vi "PathDrawerMain.vi"() -> ()   [LabVIEW 2017]
uses:
  Shared/PathFileData.ctl
  Shared/RobotNeededPathData.ctl
panel:
  in  "Tab Control":enum32{"Path", "Load/Save"}(tab)
  in  "SlowSpeed":dbl=15.0 format="%#_13g"
  in  "SlowDistanceAtEnd":dbl=12.0 format="%#_13g"
  in  "Speed/Curve":dbl=2.0 format="%#_13g"
  in  "DriveBackwards?":bool
  in  "Lookahead":dbl=13.0
  out "Points (in)":cluster{dbl, dbl}[](array[cluster])=[{14.875179340028694, 248.22955523672883}, {20.874656142200276, 248.30358846723587}, {26.874111844136586, 248.37762105138137}, {32.87350807743945, 248.45164576572313}, {38.87285031681461, 248.52564930010115}, {44.8721376174185, 248.59961966708173}, {50.87132679490307, 248.67354461649725}, {56.87033754344792, 248.74740402354425}, {62.86906734714655, 248.82116341910367}, {68.86738582507886, 248.8947700228471}, {74.8651048928512, 248.9681473786283}, {80.86193607975939, 249.04118420575625}, {86.85743425686633, 249.11371611190245}, {92.85096070503305, 249.18549244057994}, {98.84145913304778, 249.25615421906943}, {104.8276556156584, 249.32512066220386}, {110.80708687815371, 249.39160976611277}, {116.77680979233328, 249.4543515328238}, {122.73186791730424, 249.5115256430506}, {128.6649834222615, 249.56041338385793}, {134.56548779738634, 249.5969246365727}, {140.417375186257, 249.6149706245841}, {146.1966910294908, 249.60548863042237}, {151.86775390690585, 249.55495714900198}, {157.37740484291632, 249.4431992192172}, {162.64635606562646, 249.2401236836006}, {167.55632241578652, 248.9008602167623}, {172.80142342709613, 248.36924030479463}, {178.27099698643164, 247.70868036210402}, {183.89073844553332, 246.9617176111296}, {189.61066276690974, 246.15689887726526}, {195.3970009046773, 245.3134049055755}, {201.22672879119182, 244.44415649854506}, {207.08384341112958, 243.55790546653972}, {212.9567773862825, 242.6606503511154}, {218.83652869344567, 241.75660718632653}, {224.71520193237015, 240.84889249476205}, {230.58472714757215, 239.94002850052652}, {236.43555125878544, 239.03235181687802}, {242.25509137335504, 238.1283916506969}, {248.0256984324822, 237.231278977795}, {253.72180303927817, 236.34525315742894}, {259.30577066584806, 235.47634844945551}, {264.7218219756948, 234.63337048251796}, {269.8869762914892, 233.8293235417345}, {274.67764890352106, 233.08351364924852}, {278.909612625538, 232.42467718794836}]
  in  "Points":cluster{dbl, dbl}[](array[cluster])=[{40.0, 78.0}, {202.0, 76.0}, {324.0, 95.0}]
  in  "Roundedness":dbl(slide)=0.8606565656565657 scale=0.6..0.997
  in  "Length":dbl=38.5
  in  "Width":dbl=33.0
  in  "CenterRotOffset":dbl=15.5
  in  "PointSpacing":dbl=6.0 min=1.0 format="%#_13g"
  in  "Flip Path":bool
  in  "MaxVel":dbl=110.0 format="%#_13g"
  in  "MaxAccel":dbl=50.0 format="%#_13g"
  in  "StartingPosition":enum16{"1", "2", "3", "4", "No Preset"}(ring)
  in  "ExportAllToRobot":bool
  in  "LocalTempPaths":i32(listbox)
  out "standard output":string
  in  "SaveToLocal":bool
  in  "LoadFromLocal":bool
  in  "ExportToRobot":bool
  in  "LoadAllFromRobot":bool
  in  "LocalPaths":i32(listbox)=2
  out "standard error":string="NI Linux Real-Time (run mode)\n\nLog in with your NI-Auth credentials.\n\n"
  in  "LocalFileNames":string[](array[string])=["1A.txt", "1B.txt", "1C.txt", "1D.txt", "2A.txt", "2B.txt", "2C.txt", "2D.txt", "3A.txt", "3B.txt", "3C.txt", "3D.txt", "4A.txt", "4B.txt", "4C.txt", "4D.txt"]
  in  "Stop":bool
  out "Path Drawer":T1(plugin-control)
  # "Includes bumpers"
  # "INSTRUCTIONS"
  # "The red line is the path that the robot recieves. Everything else is to help create that path\n\nUse the multi-line tool to draw a path. Double click to stop drawing.\nHover over a node and press backspace to remove it.\nPress I to insert a new node (at the end of the path only, for now)\n\nUse the contols to input robot width, height, and center of rotation offset,\nHow far apart the points in the \"real world units\" path are,\nWhether the robot travels on the left or right of your green lines, and\nthe roundedness of the path. (Note: point spacing affects roundedness)\n\nYou can manually edit the green node's location in the path with the Points array,\nor drag the nodes on the image\n\nPress Export To File and enter the file name (no extension) to save the path to a file in the\nThisVIsDirectory\\Paths\\ folder\n\nIf you acidentally clear your path press Z quickly to get it back"
  # "Responses of CMDs run"
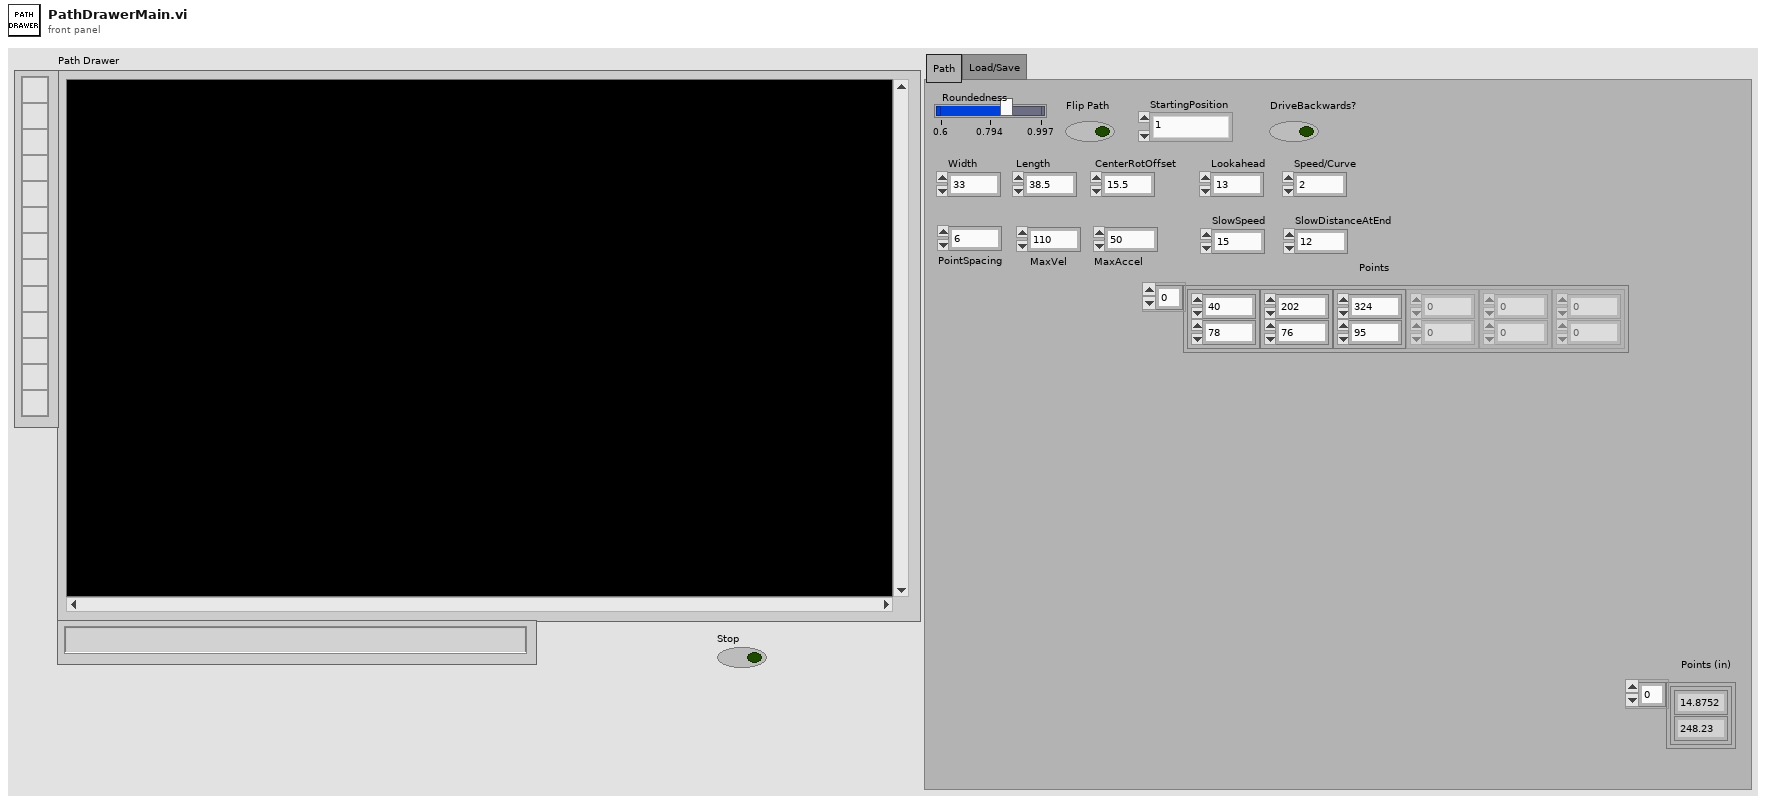
[diagram p1: front panel]
types:
  T1 = typedef "IMAQ Image.ctl" = refnum<image>
  T2 = typedef "Image Type" = u32
  T3 = enum16{"open", "replace", "create", "open or create", "replace or create", "replace or create with confirmation"}
  T4 = cluster{"Global Rectangle":i32[], "Contours":cluster{"Contour Type":u32, "ROI Type":u32, "Points":i32[]}[]}
  T5 = cluster{"Contour Type":u32, "ROI Type":u32, "Points":i32[]}[]
  T6 = cluster{"Contour Type":u32, "ROI Type":u32, "Points":i32[]}
  T7 = typedef "PathFileData.ctl" = cluster{"RobotNeeded":T8, "Meta":cluster{"Path (px)":cluster{i32, i32}[], "RobotWidth":dbl, "RobotLength":dbl, "CenterOfRotYOffset":dbl, "Roundedness":dbl, "StartingPositionPreset":u32, "PathName":string}}
  T8 = typedef "RobotNeededPathData.ctl" = cluster{"Path":cluster{dbl, dbl}[], "MaxVel":dbl, "MaxAccel":dbl, "Backwards?":bool, "PointSpacing":dbl, "LookaheadDist":dbl, "Speed/Curve":dbl, "SlowDistanceAtEnd":dbl, "SlowSpeed":dbl}
  T9 = cluster{"Path (px)":cluster{i32, i32}[], "RobotWidth":dbl, "RobotLength":dbl, "CenterOfRotYOffset":dbl, "Roundedness":dbl, "StartingPositionPreset":u32, "PathName":string}
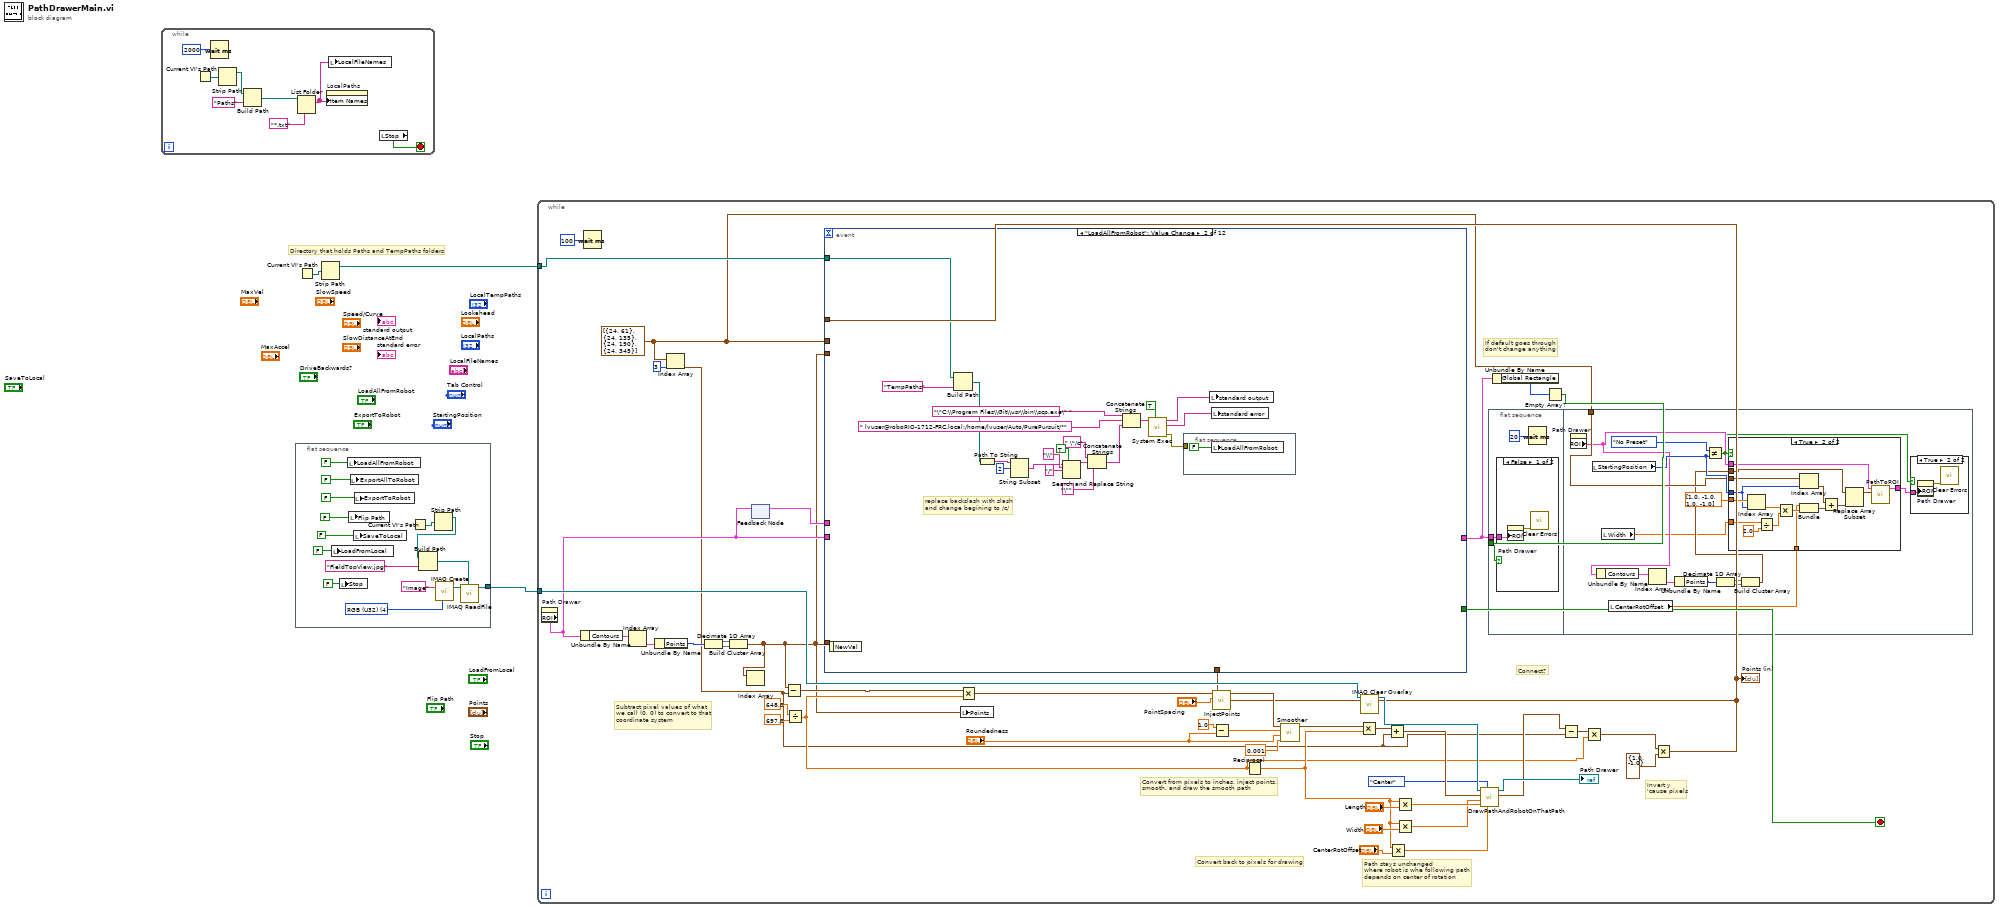
[diagram p0: block diagram]
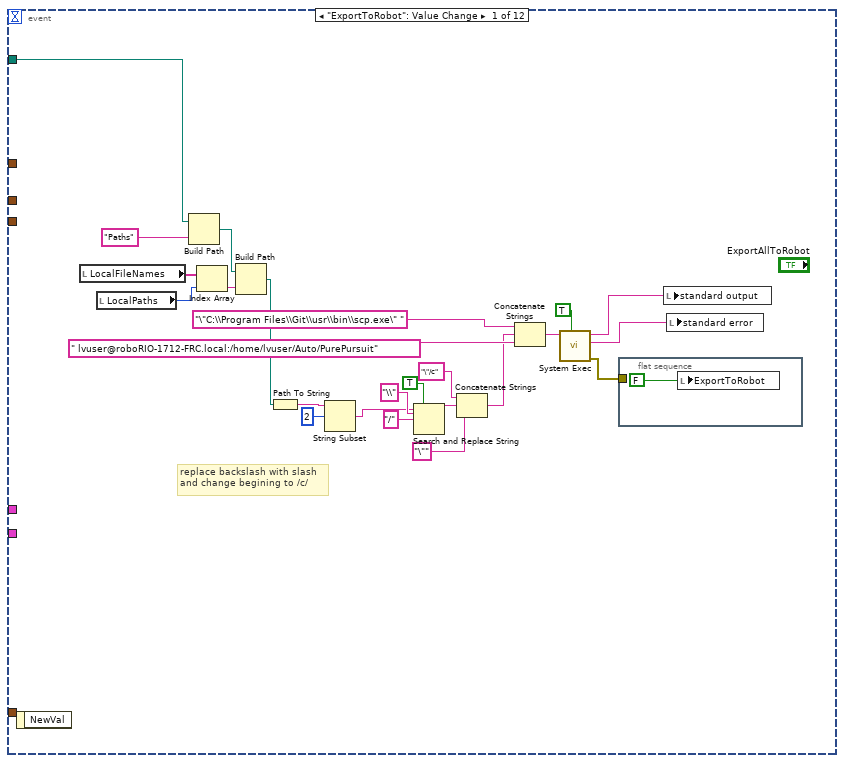
[diagram p5: hidden frame]
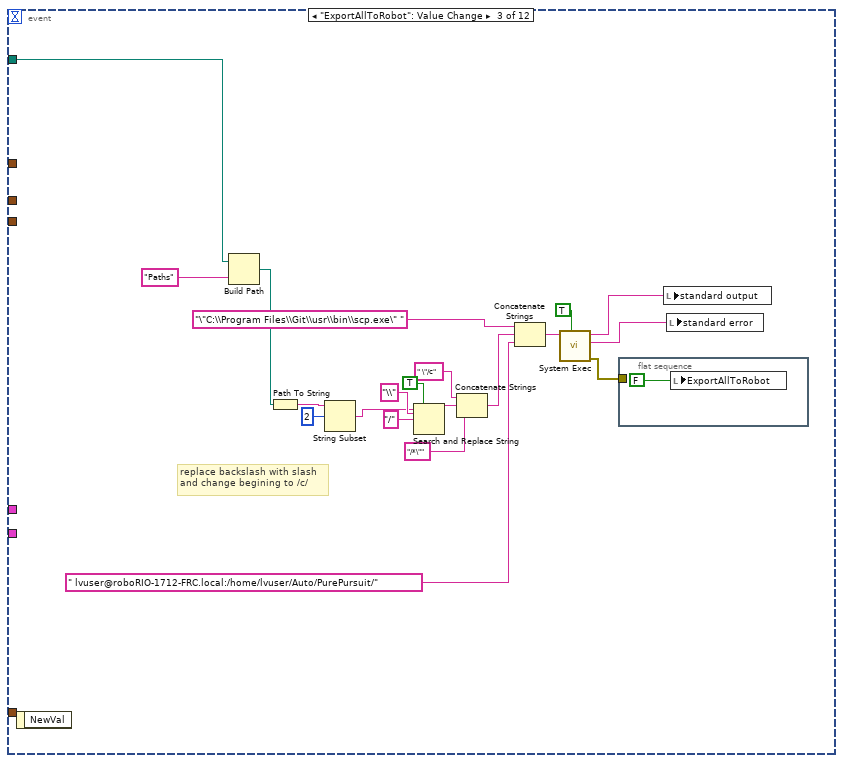
[diagram p6: hidden frame]
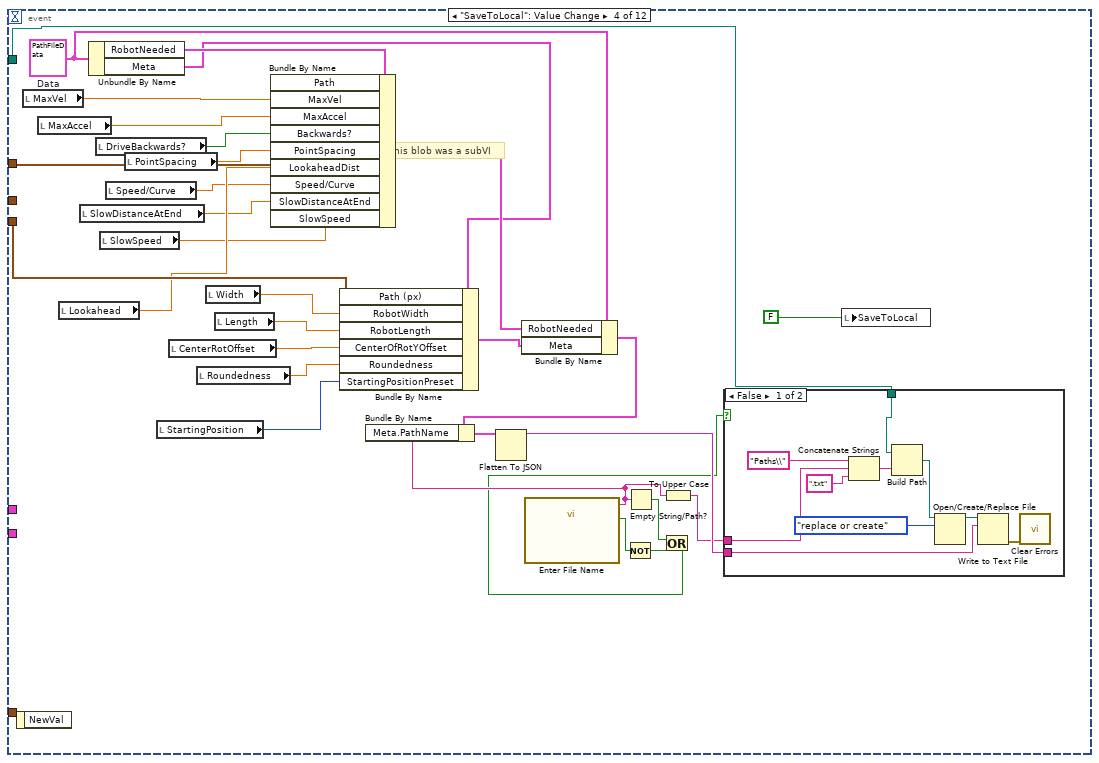
[diagram p7: hidden frame]
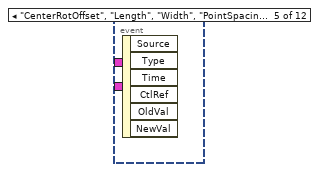
[diagram p9: hidden frame]
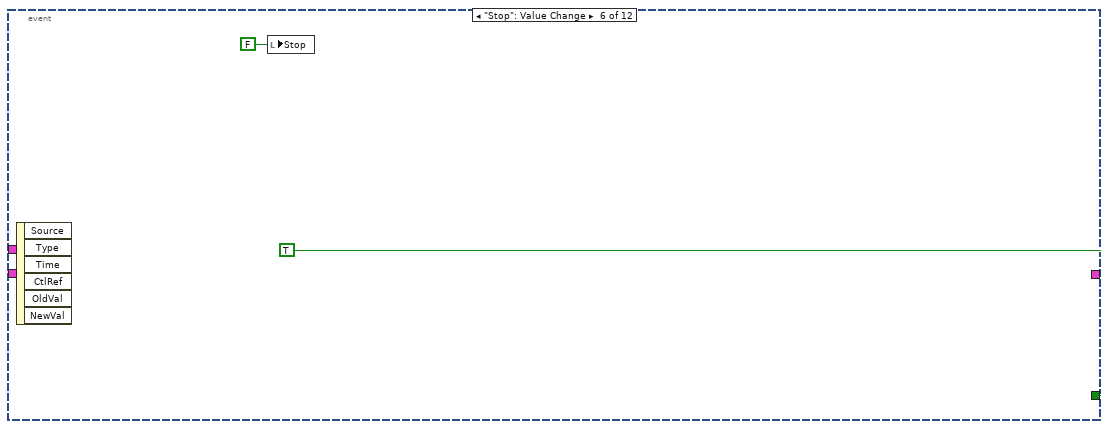
[diagram p10: hidden frame]
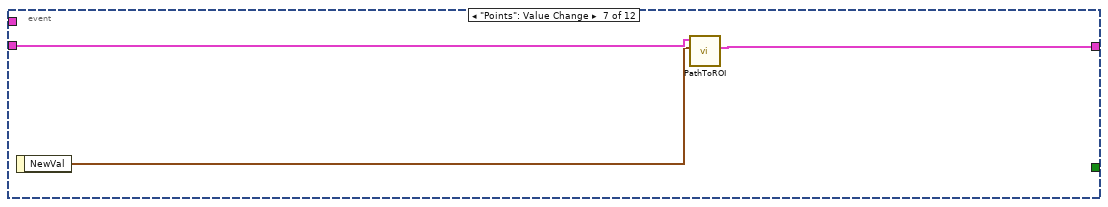
[diagram p11: hidden frame]
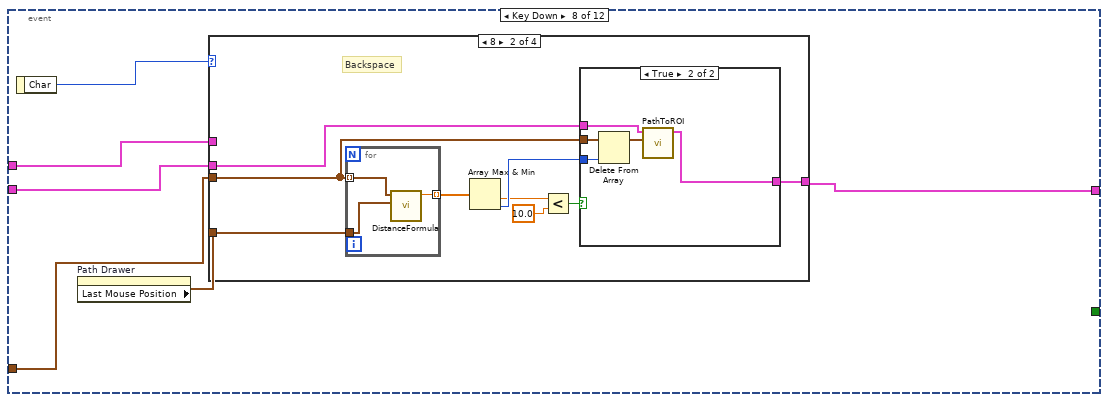
[diagram p12: hidden frame]
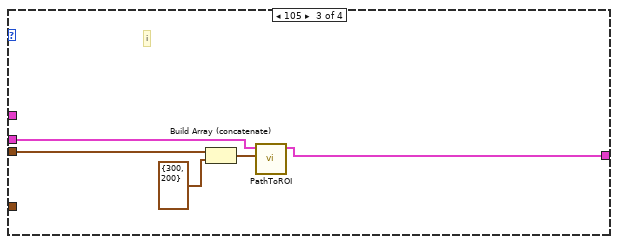
[diagram p15: hidden frame]
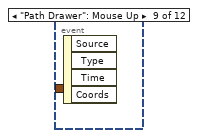
[diagram p17: hidden frame]
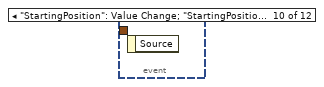
[diagram p18: hidden frame]
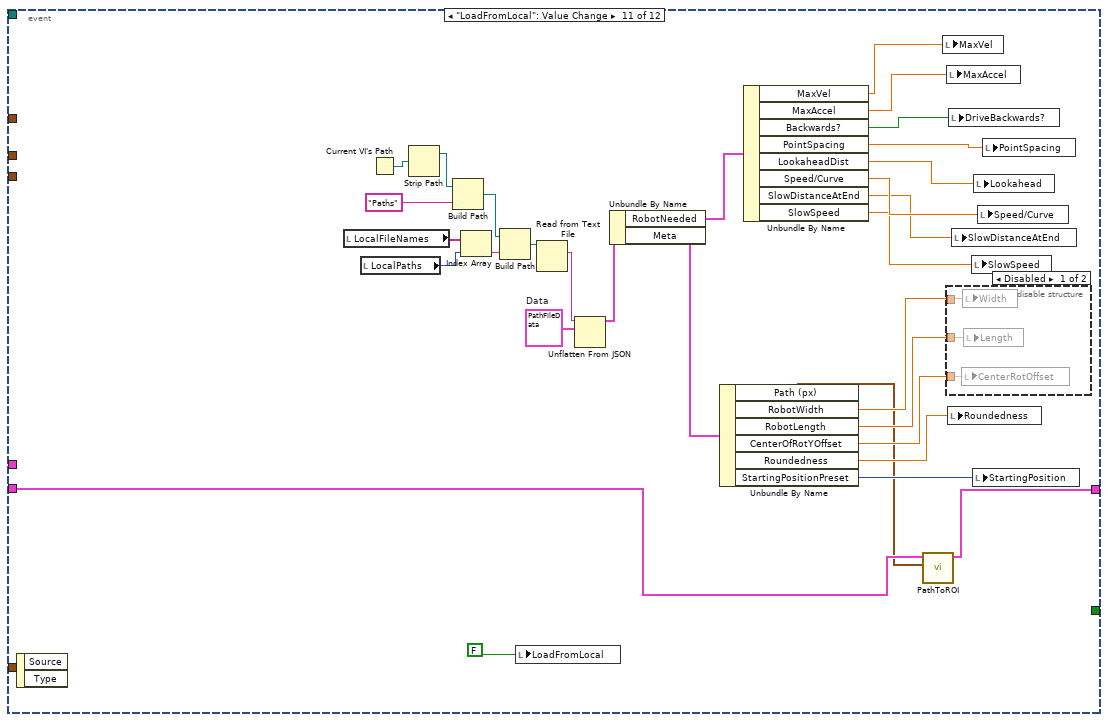
[diagram p19: hidden frame]
diagram:
  # "Directory that holds Paths and TempPaths folders"
  n1 = while {
    stop <- w10 stop-if-true
    n2 = Current VI's Path() -> (path=w5:path)
    n3 = Wait (ms)(milliseconds to wait=u32 2000) -> ()  [unwired: 1 out]
    n4 = Strip Path(path=w5) -> (stripped path=w4:path)  [unwired: 1 out]
    n5 = Build Path(base path=w4, name or relative path="Paths") -> (appended path=w7:path)
    n6 = List Folder(path=w7, pattern="*.txt") -> (filenames=w9:string[])  [unwired: 2 in, 3 out]
    n7 = property on="LocalPaths" class="LstBox (strict)"("Item Names"=w9) -> ()  [unwired: 2 in, 2 out]
    n8 = local write "LocalFileNames"(w9) -> ()
    n9 = local read "Stop"() -> (w10:bool)
  }
  n10 = flat-sequence {
    tunnel: [w21] -> w3
    frame #0 {
      w23 = T2 4 items=["Grayscale (U8)", "Grayscale (I16)", "Grayscale (SGL)", "Complex (CSG)", "RGB (U32)", "HSL (U32)", "RGB (U64)", "Grayscale (U16)"] ("Image Type")
      n11 = local write "LoadFromLocal"(FALSE ("Export To File")) -> ()
      n12 = local write "Stop"(FALSE ("Stop")) -> ()
      n13 = local write "LoadAllFromRobot"(FALSE ("Export To File")) -> ()
      n14 = local write "Flip Path"(FALSE ("Export To File")) -> ()
      n15 = local write "ExportAllToRobot"(FALSE ("Export To File")) -> ()
      n16 = local write "SaveToLocal"(FALSE ("Export To File")) -> ()
      n17 = local write "ExportToRobot"(FALSE ("Export To File")) -> ()
      n18 = Current VI's Path() -> (path=w15:path)
      n19 = Strip Path(path=w15) -> (stripped path=w14:path)  [unwired: 1 out]
      n20 = Build Path(base path=w14, name or relative path="FieldTopView.jpg") -> (appended path=w25:path)
      n21 = call "IMAQ Create"("Image Name"="Image", "Image Type"=w23) -> ("New Image"=w22:T1)  [unwired: 3 in, 1 out]
      n22 = call "IMAQ ReadFile"("File Path"=w25, "Image"=w22) -> ("Image Out"=w21:T1)  [unwired: 5 in, 4 out]
    }
  }
  n23 = Current VI's Path() -> (path=w2:path)
  n24 = Strip Path(path=w2) -> (stripped path=w1:path)  [unwired: 1 out]
  n25 = while {
    tunnel: w3 -> [w67]
    tunnel: w1 -> [w33]
    stop <- w41 stop-if-true
    w27 = cluster{i32, i32}[] [{24, 61}, {24, 135}, {24, 190}, {24, 345}]
    # "Connect?"
    # "Invert y\n'cause pixels"
    # "Path stays unchanged\nwhere robot is whe following path\ndepends on center of rotation"
    # "Convert back to pixels for drawing"
    # "If default goes through\ndon't change anything"
    # "Convert from pixels to inches, inject points,\nsmooth, and draw the smooth path"
    # "Subtract pixel values of what\nwe call (0, 0) to convert to that\ncoordinate system"
    n26 = property on="Path Drawer" class="ImageControl"() -> ("ROI"=w37:T4)  [unwired: 2 in, 2 out]
    n27 = Unbundle By Name(w37) -> ("Contours"=w73:T5)
    n28 = Wait (ms)(milliseconds to wait=u32 100) -> ()  [unwired: 1 out]
    n29 = Index Array(array=w73) -> (element=w68:T6)  [unwired: 1 in]
    n30 = Unbundle By Name(w68) -> ("Points"=w62:i32[])
    n31 = Index Array(array=w27, index=3) -> (element=w31:cluster{i32, i32})
    n32 = Decimate 1D Array(w62) -> (w72:i32[], w71:i32[])
    n33 = Build Cluster Array(w72, w71) -> (w35:cluster{i32, i32}[])
    n34 = Index Array(array=w35) -> ()  [unwired: 1 in, 1 out]
    n35 = feedback-in #1(w37) -> ()
    n36 = feedback #1() -> (w50:T4)  [unwired: 1 in]
    n37 = Subtract(x=w35, y=w31) -> (x-y=w63:cluster{i32, i32}[])
    n38 = Divide(x=648.0, y=697.0) -> (x/y=w38:dbl)
    n39 = Multiply(x=w63, y=w38) -> (x*y=w51:cluster{dbl, dbl}[])
    n40 = local write "Points"(w35) -> ()
    n41 = call "InjectPoints.vi"("Distance"="PointSpacing", "Path"=w51) -> ("Path out"=w65:cluster{dbl, dbl}[])  [unwired: 9 in]
    n42 = Subtract(x=1.0, y="Roundedness") -> (x-y=w60:dbl)
    n43 = Reciprocal(x=w38) -> (1/x=w48:dbl)
    n44 = call "Smoother.vi"("tolerance"=0.001, "B"="Roundedness", "A"=w60, "Path"=w65) -> ("SmoothPath"=w56:cluster{dbl, dbl}[])  [unwired: 7 in]
    n45 = Multiply(x=w56, y=w48) -> (x*y=w64:cluster{dbl, dbl}[])
    n46 = call "IMAQ Clear Overlay"("Image"=w67) -> ("Image Out"=w45:T1)  [unwired: 9 in, 1 out]
    n47 = Add(x=w64, y=w31) -> (x+y=w44:cluster{dbl, dbl}[])
    n48 = Multiply(x=w48, y="CenterRotOffset") -> (x*y=w28:dbl)
    n49 = Multiply(x=w48, y="Length") -> (x*y=w43:dbl)
    n50 = Multiply(x=w48, y="Width") -> (x*y=w29:dbl)
    n51 = call "DrawPathAndRobotOnThatPath.vi"("CenterOfRotYOffset (px)"=w28, "PathMode"=enum16{"Left", "Right", "Center"}."Center", "RobotLength (px)"=w43, "RobotWidth (px)"=w29, "Path (px)"=w44, "Image In"=w45) -> ("NewPath (px)"=w46:cluster{dbl, dbl}[], "Image Out"=→"Path Drawer":T1)  [unwired: 4 in]
    n52 = flat-sequence {
      tunnel: w36 -> [w76]
      tunnel: w30 -> [w75]
      tunnel: w27 -> [w90]
      frame #0 {
        n53 = case shown="False" w75 {
          tunnel: w76 -> [w77 _]
          frame False {
            n54 = property on="Path Drawer" class="ImageControl"("ROI"=w77) -> (error out=w78:errorcluster)  [unwired: 2 in, 1 out]
            n55 = call <vilib>:"Clear Errors.vi"("error in (no error)"=w78) -> ()  [unwired: 5 in, 2 out]
          }
          frame True {
          }
        }
        n56 = Wait (ms)(milliseconds to wait=u32 20) -> ()  [unwired: 1 out]
      }
      frame #1 {
        n57 = property on="Path Drawer" class="ImageControl"() -> ("ROI"=w84:T4)  [unwired: 2 in, 2 out]
        n58 = local read "StartingPosition"() -> (w91:enum16{"1", "2", "3", "4", "No Preset"})
        n59 = Unbundle By Name(w84) -> ("Contours"=w85:T5)
        n60 = local read "Width"() -> (w80:dbl)
        n61 = local read "CenterRotOffset"() -> (w79:dbl)
        n62 = Index Array(array=w85) -> (element=w88:T6)  [unwired: 1 in]
        n63 = Unbundle By Name(w88) -> ("Points"=w89:i32[])
        n64 = Not Equal?(x=enum16{"1", "2", "3", "4", "No Preset"}."No Preset" ("y"), y=w91) -> (x != y?=w81:bool)
        n65 = Decimate 1D Array(w89) -> (w86:i32[], w87:i32[])
        n66 = Build Cluster Array(w86, w87) -> (w83:cluster{i32, i32}[])
        n67 = case shown="True" w81 {
          tunnel: [_ w111] -> w82
          tunnel: w84 -> [_ w110]
          tunnel: w83 -> [_ w108]
          tunnel: w91 -> [_ w98]
          tunnel: w80 -> [_ w102]
          tunnel: w90 -> [_ w101]
          tunnel: dbl[] [1.0, -1.0, 1.0, -1.0] -> [_ w99]
          tunnel: w79 -> [_ w96]
          frame False {
          }
          frame True {
            n68 = Index Array(array=w99, index=w98) -> (element=w97:dbl)
            n69 = Divide(x=w102, y=2.0) -> (x/y=w105:dbl)
            n70 = Multiply(x=w97, y=w105) -> (x*y=w104:dbl)
            n71 = Index Array(array=w101, index=w98) -> (element=w100:cluster{i32, i32})
            n72 = Bundle("CenterRotOffset"=w96, w104) -> (w103:cluster{"CenterRotOffset":dbl, dbl})  [unwired: 1 in]
            n73 = Add(x=w100, y=w103) -> (x+y=w107:cluster{dbl, dbl})
            n74 = Replace Array Subset(array=w108, new element=w107) -> (w109:cluster{i32, i32}[])  [unwired: 1 in]
            n75 = call "PathToROI.vi"("Path In"=w109, "ROI In"=w110) -> ("ROI Out"=w111:T4)  [unwired: 9 in]
          }
        }
        n76 = case shown="True" w81 {
          tunnel: w82 -> [_ w94]
          frame False {
          }
          frame True {
            n77 = property on="Path Drawer" class="ImageControl"("ROI"=w94) -> (error out=w95:errorcluster)  [unwired: 2 in, 1 out]
            n78 = call <vilib>:"Clear Errors.vi"("error in (no error)"=w95) -> ()  [unwired: 5 in, 2 out]
          }
        }
      }
    }
    n79 = Subtract(x=w46, y=w31) -> (x-y=w52:cluster{dbl, dbl}[])
    n80 = Multiply(x=w52, y=w38) -> (x*y=w40:cluster{dbl, dbl}[])
    n81 = Multiply(x=w40, y=cluster{dbl, dbl} {1.0, -1.0}) -> (x*y=w34:cluster{dbl, dbl}[])
    "Points (in)" <- w34
    n82 = event shown="[1] \"LoadAllFromRobot\": Value Change" {
      selector: _ -> [_ _ _ _ _ _ _ _ _ _ _ _]
      dyn-events: _ -> [_ _ _ _ _ _ _ _ _ _ _ _]
      timeout: _ -> [_ _ _ _ _ _ _ _ _ _ _ _]
      tunnel: w37 -> [_ _ _ _ _ _ w224 w230 _ _ w270 w300]
      tunnel: [_ _ _ _ _ _ w223 w227 _ _ w284 w299] -> w36
      tunnel: w34 -> [_ _ _ _ _ _ _ _ _ _ _ _]
      tunnel: w50 -> [_ _ _ _ _ _ _ w226 _ _ _ _]
      tunnel: w35 -> [_ _ _ _ _ _ _ w225 _ _ _ w294]
      tunnel: [_ _ _ _ _ TRUE ("Stop") _ _ _ _ _ _] -> w41
      tunnel: w35 -> [_ _ _ w193 _ _ _ _ _ _ _ _]
      tunnel: w34 -> [_ _ _ w192 _ _ _ _ _ _ _ _]
      tunnel: w33 -> [w112 w137 w158 w185 _ _ _ _ _ _ _ _]
      tunnel: w27 -> [_ _ _ _ _ _ _ _ _ _ _ _]
      event "ExportToRobot": Value Change {
        # "replace backslash with slash\nand change begining to /c/"
        n83 = event-data() -> ()  [unwired: 1 in, 1 out]
        n84 = local read "LocalFileNames"() -> (w119:string[])
        n85 = local read "LocalPaths"() -> (w120:i32)
        n86 = Build Path(base path=w112, name or relative path="Paths") -> (appended path=w122:path)
        n87 = Index Array(array=w119, index=w120) -> (element=w121:string)
        n88 = Build Path(base path=w122, name or relative path=w121) -> (appended path=w117:path)
        n89 = Path To String(path=w117) -> (string=w128:string)
        n90 = String Subset(string=w128, offset (0)=2) -> (substring=w126:string)  [unwired: 1 in]
        n91 = Search and Replace String(replace all?=TRUE ("replace all? (F)"), input string=w126, search string="\\", replace string="/" ("replace string (\"\")")) -> (result string=w125:string)  [unwired: 4 in, 3 out]
        n92 = Concatenate Strings("\"/c" ("string"), w125, "\"" ("string")) -> (w123:string)
        n93 = Concatenate Strings("\"C:\\Program Files\\Git\\usr\\bin\\scp.exe\" " ("command line"), w123, " lvuser@roboRIO-1712-FRC.local:/home/lvuser/Auto/PurePursuit" ("string")) -> (w132:string)
        n94 = call <vilib>:"System Exec.vi"("wait until completion? (T)"=TRUE, "command line"=w132) -> ("error out"=w115:errorcluster, "standard error"=w113:string, "standard output"=w114:string)  [unwired: 6 in, 1 out]
        n95 = flat-sequence {
          tunnel: w115 -> [_]
          frame #0 {
            n96 = local write "ExportToRobot"(FALSE ("Export To File")) -> ()
          }
        }
        n97 = local write "standard output"(w114) -> ()
        n98 = local write "standard error"(w113) -> ()
      }
      event "LoadAllFromRobot": Value Change {
        # "replace backslash with slash\nand change begining to /c/"
        n99 = event-data() -> ()  [unwired: 1 in, 1 out]
        n100 = Build Path(base path=w137, name or relative path="TempPaths") -> (appended path=w140:path)
        n101 = Path To String(path=w140) -> (string=w150:string)
        n102 = String Subset(string=w150, offset (0)=2) -> (substring=w148:string)  [unwired: 1 in]
        n103 = Search and Replace String(replace all?=TRUE ("replace all? (F)"), input string=w148, search string="\\", replace string="/" ("replace string (\"\")")) -> (result string=w147:string)  [unwired: 4 in, 3 out]
        n104 = Concatenate Strings(" \"/c" ("string"), w147, "\"" ("string")) -> (w138:string)
        n105 = Concatenate Strings("\"C:\\Program Files\\Git\\usr\\bin\\scp.exe\" " ("command line"), " lvuser@roboRIO-1712-FRC.local:/home/lvuser/Auto/PurePursuit/*" ("string"), w138) -> (w154:string)
        n106 = call <vilib>:"System Exec.vi"("wait until completion? (T)"=TRUE, "command line"=w154) -> ("error out"=w143:errorcluster, "standard error"=w141:string, "standard output"=w142:string)  [unwired: 6 in, 1 out]
        n107 = flat-sequence {
          tunnel: w143 -> [_]
          frame #0 {
            n108 = local write "LoadAllFromRobot"(FALSE ("Export To File")) -> ()
          }
        }
        n109 = local write "standard output"(w142) -> ()
        n110 = local write "standard error"(w141) -> ()
      }
      event "ExportAllToRobot": Value Change {
        # "replace backslash with slash\nand change begining to /c/"
        n111 = event-data() -> ()  [unwired: 1 in, 1 out]
        n112 = Build Path(base path=w158, name or relative path="Paths") -> (appended path=w161:path)
        n113 = Path To String(path=w161) -> (string=w171:string)
        n114 = String Subset(string=w171, offset (0)=2) -> (substring=w169:string)  [unwired: 1 in]
        n115 = Search and Replace String(replace all?=TRUE ("replace all? (F)"), input string=w169, search string="\\", replace string="/" ("replace string (\"\")")) -> (result string=w168:string)  [unwired: 4 in, 3 out]
        n116 = Concatenate Strings(" \"/c" ("string"), w168, "/*\"" ("string")) -> (w160:string)
        n117 = Concatenate Strings("\"C:\\Program Files\\Git\\usr\\bin\\scp.exe\" " ("command line"), w160, " lvuser@roboRIO-1712-FRC.local:/home/lvuser/Auto/PurePursuit/" ("string")) -> (w175:string)
        n118 = call <vilib>:"System Exec.vi"("wait until completion? (T)"=TRUE, "command line"=w175) -> ("error out"=w164:errorcluster, "standard error"=w162:string, "standard output"=w163:string)  [unwired: 6 in, 1 out]
        n119 = flat-sequence {
          tunnel: w164 -> [_]
          frame #0 {
            n120 = local write "ExportAllToRobot"(FALSE ("Export To File")) -> ()
          }
        }
        n121 = local write "standard output"(w163) -> ()
        n122 = local write "standard error"(w162) -> ()
      }
      event "SaveToLocal": Value Change {
        w191 = T7 {"RobotNeeded"={"Path"=[], "MaxVel"=0.0, "MaxAccel"=0.0, "Backwards?"=FALSE, "PointSpacing"=0.0, "LookaheadDist"=0.0, "Speed/Curve"=1.8, "SlowDistanceAtEnd"=12.0, "SlowSpeed"=15.0}, "Meta"={"Path (px)"=[], "RobotWidth"=0.0, "RobotLength"=0.0, "CenterOfRotYOffset"=0.0, "Roundedness"=0.0, "StartingPositionPreset"=2, "PathName"=""}}  # Data
        # "I wish this blob was a subVI"
        n123 = event-data() -> ()  [unwired: 1 in, 1 out]
        n124 = local read "MaxVel"() -> (w184:dbl)
        n125 = local read "MaxAccel"() -> (w183:dbl)
        n126 = local read "Lookahead"() -> (w187:dbl)
        n127 = local read "SlowDistanceAtEnd"() -> (w180:dbl)
        n128 = Unbundle By Name(w191) -> ("RobotNeeded"=w200:T8, "Meta"=w199:T9)
        n129 = local read "DriveBackwards?"() -> (w186:bool)
        n130 = local read "SlowSpeed"() -> (w179:dbl)
        n131 = local read "Speed/Curve"() -> (w181:dbl)
        n132 = local read "PointSpacing"() -> (w203:dbl)
        n133 = local read "StartingPosition"() -> (w202:enum16{"1", "2", "3", "4", "No Preset"})
        n134 = local read "CenterRotOffset"() -> (w195:dbl)
        n135 = local read "Roundedness"() -> (w194:dbl)
        n136 = local read "Width"() -> (w197:dbl)
        n137 = local read "Length"() -> (w196:dbl)
        n138 = Bundle By Name(cluster=w200, "Path"=w192, "MaxVel"=w184, "MaxAccel"=w183, "Backwards?"=w186, "PointSpacing"=w203, "LookaheadDist"=w187, "Speed/Curve"=w181, "SlowDistanceAtEnd"=w180, "SlowSpeed"=w179) -> (w201:T8)
        n139 = Bundle By Name(cluster=w199, "Path (px)"=w193, "RobotWidth"=w197, "RobotLength"=w196, "CenterOfRotYOffset"=w195, "Roundedness"=w194, "StartingPositionPreset"=w202) -> (w198:T9)
        n140 = Bundle By Name(cluster=w191, "RobotNeeded"=w201, "Meta"=w198) -> (w190:T7)
        n141 = call "Enter File Name"() -> ("File Name"=w189:string, "Enter"=w205:bool)  [unwired: 17 in, 1 out]
        n142 = Bundle By Name(cluster=w190, "Meta.PathName"=w189) -> (w207:T7)
        n143 = Flatten To JSON(anything=w207) -> (JSON string=w208:string)  [unwired: 2 in, 1 out]
        n144 = Not(x=w205) -> (.not. x?=w204:bool)
        n145 = Empty String/Path?(string/path=w189) -> (empty?=w206:bool)
        n146 = Or(x=w206, y=w204) -> (x .or. y?=w182:bool)
        n147 = To Upper Case(1:w189) -> (0:w188:string)
        n148 = case shown="False" w182 {
          tunnel: w188 -> [w215 _]
          tunnel: w208 -> [w214 _]
          tunnel: w185 -> [w210 _]
          frame False {
            n149 = Concatenate Strings("Paths\\" ("name or relative path"), w215, ".txt" ("string")) -> (w219:string)
            n150 = Build Path(base path=w210, name or relative path=w219) -> (appended path=w213:path)
            n151 = Open/Create/Replace File(file path (use dialog)=w213, operation (0:open)=T3."replace or create") -> (refnum out=w212:refnum<file>)  [unwired: 4 in, 2 out]
            n152 = Write to Text File(file (use dialog)=w212, text=w214) -> (error out=w217:errorcluster)  [unwired: 2 in, 2 out]
            n153 = call <vilib>:"Clear Errors.vi"("error in (no error)"=w217) -> ()  [unwired: 5 in, 2 out]
          }
          frame True {
          }
        }
        n154 = local write "SaveToLocal"(FALSE ("Export To File")) -> ()
      }
      event "CenterRotOffset", "Length", "Width", "PointSpacing", "Roundedness": Value Change {
        n155 = event-data() -> ()  [unwired: 1 in, 6 out]
      }
      event "Stop": Value Change {
        n156 = event-data() -> ()  [unwired: 1 in, 6 out]
        n157 = local write "Stop"(FALSE ("Stop")) -> ()
      }
      event "Points": Value Change {
        n158 = event-data() -> ("NewVal"=w222:cluster{dbl, dbl}[])  [unwired: 1 in]
        n159 = call "PathToROI.vi"("Path In"=w222, "ROI In"=w224) -> ("ROI Out"=w223:T4)  [unwired: 9 in]
      }
      event Key Down {
        n160 = event-data() -> ("Char"=w229:i16)  [unwired: 1 in]
        n161 = property on="Path Drawer" class="ImageControl"() -> ("Last Mouse Position"=w228:cluster{"X":i32, "Y":i32})  [unwired: 2 in, 2 out]
        n162 = case shown="8" w229 {
          tunnel: w230 -> [w231 w240 w252 _]
          tunnel: w225 -> [_ w239 w254 _]
          tunnel: w228 -> [_ w233 _ _]
          tunnel: [w231 w232 w250 w255] -> w227
          tunnel: w226 -> [_ _ _ w255]
          frame 0, Default {
          }
          frame 8 {
            # "Backspace"
            n163 = for {
              tunnel: w239 -> [w249] mode=indexing
              tunnel: [w248] -> w238 mode=indexing
              tunnel: w233 -> [w247]
              n164 = call "DistanceFormula.vi"("Point 2"=w247, "Point 1"=w249) -> ("Distance"=w248:dbl)  [unwired: 9 in]
            }
            n165 = Array Max & Min(array=w238) -> (min value=w236:dbl, min index (indices)=w237:i32)  [unwired: 2 out]
            n166 = Less?(x=w236, y=10.0) -> (x < y?=w234:bool)
            n167 = case shown="True" w234 {
              tunnel: w237 -> [_ w246]
              tunnel: w239 -> [_ w245]
              tunnel: w240 -> [w241 w243]
              tunnel: [w241 w242] -> w232
              frame False {
              }
              frame True {
                n168 = Delete From Array(array=w245, index=w246) -> (array with subset deleted=w244:cluster{i32, i32}[])  [unwired: 1 in, 1 out]
                n169 = call "PathToROI.vi"("Path In"=w244, "ROI In"=w243) -> ("ROI Out"=w242:T4)  [unwired: 9 in]
              }
            }
          }
          frame 105 {
            # "i"
            n170 = Build Array (concatenate)(w254, cluster{i32, i32} {300, 200}) -> (w253:cluster{i32, i32}[])
            n171 = call "PathToROI.vi"("Path In"=w253, "ROI In"=w252) -> ("ROI Out"=w250:T4)  [unwired: 9 in]
          }
          frame 122 {
            # "Restore last ROI"
            # "Z"
          }
        }
      }
      event "Path Drawer": Mouse Up {
        n172 = event-data() -> ()  [unwired: 1 in, 4 out]
      }
      event "StartingPosition": Value Change; "StartingPosition": Mouse Down {
        n173 = event-data() -> ()  [unwired: 1 in, 1 out]
      }
      event "LoadFromLocal": Value Change {
        w281 = T7 {"RobotNeeded"={"Path"=[], "MaxVel"=0.0, "MaxAccel"=0.0, "Backwards?"=FALSE, "PointSpacing"=0.0, "LookaheadDist"=0.0, "Speed/Curve"=1.8, "SlowDistanceAtEnd"=12.0, "SlowSpeed"=15.0}, "Meta"={"Path (px)"=[], "RobotWidth"=0.0, "RobotLength"=0.0, "CenterOfRotYOffset"=0.0, "Roundedness"=0.0, "StartingPositionPreset"=2, "PathName"=""}}  # Data
        n174 = event-data() -> ()  [unwired: 1 in, 2 out]
        n175 = local read "LocalFileNames"() -> (w265:string[])
        n176 = local read "LocalPaths"() -> (w266:i32)
        n177 = Current VI's Path() -> (path=w268:path)
        n178 = Strip Path(path=w268) -> (stripped path=w267:path)  [unwired: 1 out]
        n179 = Build Path(base path=w267, name or relative path="Paths") -> (appended path=w273:path)
        n180 = Index Array(array=w265, index=w266) -> (element=w272:string)
        n181 = Build Path(base path=w273, name or relative path=w272) -> (appended path=w271:path)
        n182 = local write "LoadFromLocal"(FALSE ("Export To File")) -> ()
        n183 = Read from Text File(file (use dialog)=w271) -> (text=w283:string)  [unwired: 3 in, 3 out]
        n184 = Unflatten From JSON(JSON string=w283, type and defaults=w281) -> (value=w280:T7)  [unwired: 5 in, 1 out]
        n185 = Unbundle By Name(w280) -> ("RobotNeeded"=w264:T8, "Meta"=w279:T9)
        n186 = Unbundle By Name(w279) -> ("Path (px)"=w269:cluster{i32, i32}[], "RobotWidth"=w274:dbl, "RobotLength"=w275:dbl, "CenterOfRotYOffset"=w278:dbl, "Roundedness"=w277:dbl, "StartingPositionPreset"=w276:u32)
        n187 = Unbundle By Name(w264) -> ("MaxVel"=w263:dbl, "MaxAccel"=w262:dbl, "Backwards?"=w261:bool, "PointSpacing"=w260:dbl, "LookaheadDist"=w259:dbl, "Speed/Curve"=w258:dbl, "SlowDistanceAtEnd"=w257:dbl, "SlowSpeed"=w256:dbl)
        n188 = call "PathToROI.vi"("Path In"=w269, "ROI In"=w270) -> ("ROI Out"=w284:T4)  [unwired: 9 in]
        n189 = local write "MaxVel"(w263) -> ()
        n190 = local write "MaxAccel"(w262) -> ()
        n191 = disable-structure shown="Disabled" {
          disable-tunnel: w278 -> [w288 _]
          disable-tunnel: w275 -> [w287 _]
          disable-tunnel: w274 -> [w286 _]
          frame Disabled {
            n192 = local write "CenterRotOffset"(w288) -> ()
            n193 = local write "Width"(w286) -> ()
            n194 = local write "Length"(w287) -> ()
          }
          frame Enabled {
          }
        }
        n195 = local write "Roundedness"(w277) -> ()
        n196 = local write "DriveBackwards?"(w261) -> ()
        n197 = local write "SlowDistanceAtEnd"(w257) -> ()
        n198 = local write "SlowSpeed"(w256) -> ()
        n199 = local write "StartingPosition"(w276) -> ()
        n200 = local write "Lookahead"(w259) -> ()
        n201 = local write "Speed/Curve"(w258) -> ()
        n202 = local write "PointSpacing"(w260) -> ()
      }
      event "Flip Path": Value Change {
        w296 = cluster{i32, i32} {0, 203}
        # "Center of field"
        n203 = event-data() -> ()  [unwired: 1 in, 2 out]
        n204 = local read "StartingPosition"() -> (w290:enum16{"1", "2", "3", "4", "No Preset"})
        n205 = local write "Flip Path"(FALSE ("Export To File")) -> ()
        n206 = Not Equal?(x=enum16{"1", "2", "3", "4", "No Preset"}."No Preset", y=w290) -> (x != y?=w291:bool)
        n207 = Subtract(x=w294, y=w296) -> (x-y=w295:cluster{i32, i32}[])
        n208 = case shown="True" w291 {
          tunnel: w290 -> [w302 w305]
          tunnel: [w302 w303] -> w289
          frame False {
          }
          frame True {
            n209 = Subtract(x=3, y=w305) -> (x-y=w303:i32)
          }
        }
        n210 = Multiply(x=w295, y=cluster{i32, i32} {1, -1}) -> (x*y=w297:cluster{i32, i32}[])
        n211 = Add(x=w297, y=w296) -> (x+y=w293:cluster{i32, i32}[])
        n212 = call "PathToROI.vi"("Path In"=w293, "ROI In"=w300) -> ("ROI Out"=w299:T4)  [unwired: 9 in]
        n213 = local write "StartingPosition"(w289) -> ()
      }
    }
    n214 = Unbundle By Name(w36) -> ("Global Rectangle"=w57:i32[])
    n215 = Empty Array?(array=w57) -> (empty?=w30:bool)
  }
